vi "test_definitions_module.vi"() -> ()   [LabVIEW 2015]
panel:
  out "Total test time":dbl format="%.2f"
  out "overlap":dbl format="%.2f"
  out "String":string
  in  "Delay":dbl
  out "19572 Total time":dbl format="%.2f"
  out "19052 Total time":dbl format="%.2f"
  in  "VISA resource in 19572":refnum<visa-resource-name>
  in  "VISA resource in 19052":refnum<visa-resource-name>
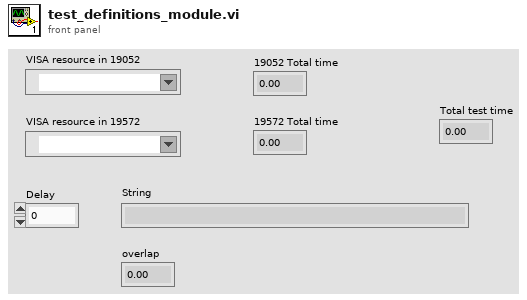
[diagram p1: front panel]
types:
  T1 = cluster{"steps":u16[], "times":string[], "active steps":u16, "modes":string[], "Total time":dbl, "CONT.?":bool}
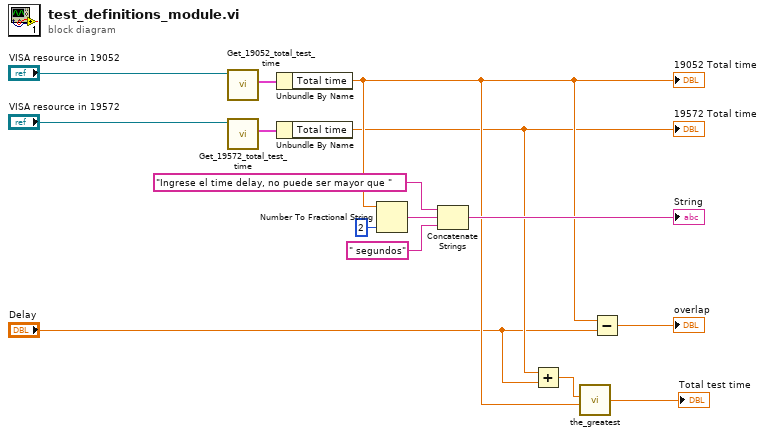
[diagram p0: block diagram]
diagram:
  n1 = call "Get_19052_total_test_time.vi"("VISA resource in"="VISA resource in 19052") -> ("Data"=w12:T1)  [unwired: 8 in, 2 out]
  n2 = call "Get_19572_total_test_time.vi"("VISA resource in"="VISA resource in 19572") -> ("Data"=w13:T1)  [unwired: 8 in, 2 out]
  n3 = Unbundle By Name(w12) -> ("Total time"=w6:dbl)
  "19052 Total time" <- w6
  n4 = Unbundle By Name(w13) -> ("Total time"=w3:dbl)
  "19572 Total time" <- w3
  n5 = Number To Fractional String(number=w6, precision (6)=i16 2) -> (F-format string=w10:string)  [unwired: 2 in]
  n6 = Concatenate Strings("Ingrese el time delay, no puede ser mayor que ", w10, " segundos") -> (→"String":string)
  n7 = Add(x=w3, y="Delay") -> (x+y=w1:dbl)
  n8 = call "the_greatest.vi"("A"=w1, "B"=w6) -> ("Greatest"=→"Total test time":dbl)  [unwired: 6 in]
  n9 = Subtract(x=w6, y="Delay") -> (x-y=→"overlap":dbl)
